vi "Calculate Source Voltage Array.vi"(8 "error in":errorcluster, 11 "measurement configuration":T1={"Mode of operation"=enum."Perform measurement", "DUT setup time"=1.0, "Source delay"=0.005, "Aperture time"=0.005, "Nominal output voltage"=3.3, "Source pin name array"=[], "Source pin name index for efficiency"=0, "Source sense array"=[], "Source current limit array"=[], "Source maximum power array"=[], "Source start voltage array"=[], "Source stop voltage array"=[], "Source voltage sweep points"=10, "Use Source voltage array"=FALSE, "Source voltage concatenated array"=[], "Source voltage array size"=[], "Load pin name"="", "Load sense"=1009, "Load voltage limit range"=6.0, "Load sweep type"="Logarithmic", "Load start current"=0.1, "Load stop current"=24.0, "Load current sweep points/points per decade"=10, "Use Load current array"=FALSE, "Load current array"=[], "Pin Names for Scope"=[], "vertical range"=[], "vertical offset"=[], "probe attenuation"=[], "vertical coupling"=[], "channel enabled"=[], "input impedance"=[], "max input frequency"=[], "min sample rate"=[], "reference position"=[], "min record length"=[], "enforce realtime"=[], "dmm pin names"=[], "dmm function array"=[], "dmm resolution in digits array"=[], "dmm range array"=[]} {"Source sense array" items=["Local"=1008, "Remote"=1009]; "dmm resolution in digits array" items=["3 1/2"=3.5, "4 1/2"=4.5, "5 1/2"=5.5, "6 1/2"=6.5, "7 1/2"=7.5]; "input impedance" items=["1 mega ohm"=0, "50 ohms"=2]; "vertical coupling" items=["AC", "DC", "Ground"]; "Load sense" items=["Local"=1008, "Remote"=1009]}) -> (0 "error out":errorcluster, 2 "Source voltage array size":i32[](array[numeric]), 3 "Source voltage array":dbl[][](array[numeric]))   [LabVIEW 2021, in "Efficiency And Load Regulation with Pin Map.lvlib"]
uses:
  Efficiency And Load Regulation with Pin Map.lvlib
  Measurement Configuration.ctl
  <instrlib>/niScope/Controls/niScope vertical coupling.ctl
  <instrlib>/niDMM/nidmm.llb/niDMM Function.ctl
  <instrlib>/niDMM/nidmm.llb/niDMM Resolution in Digits.ctl
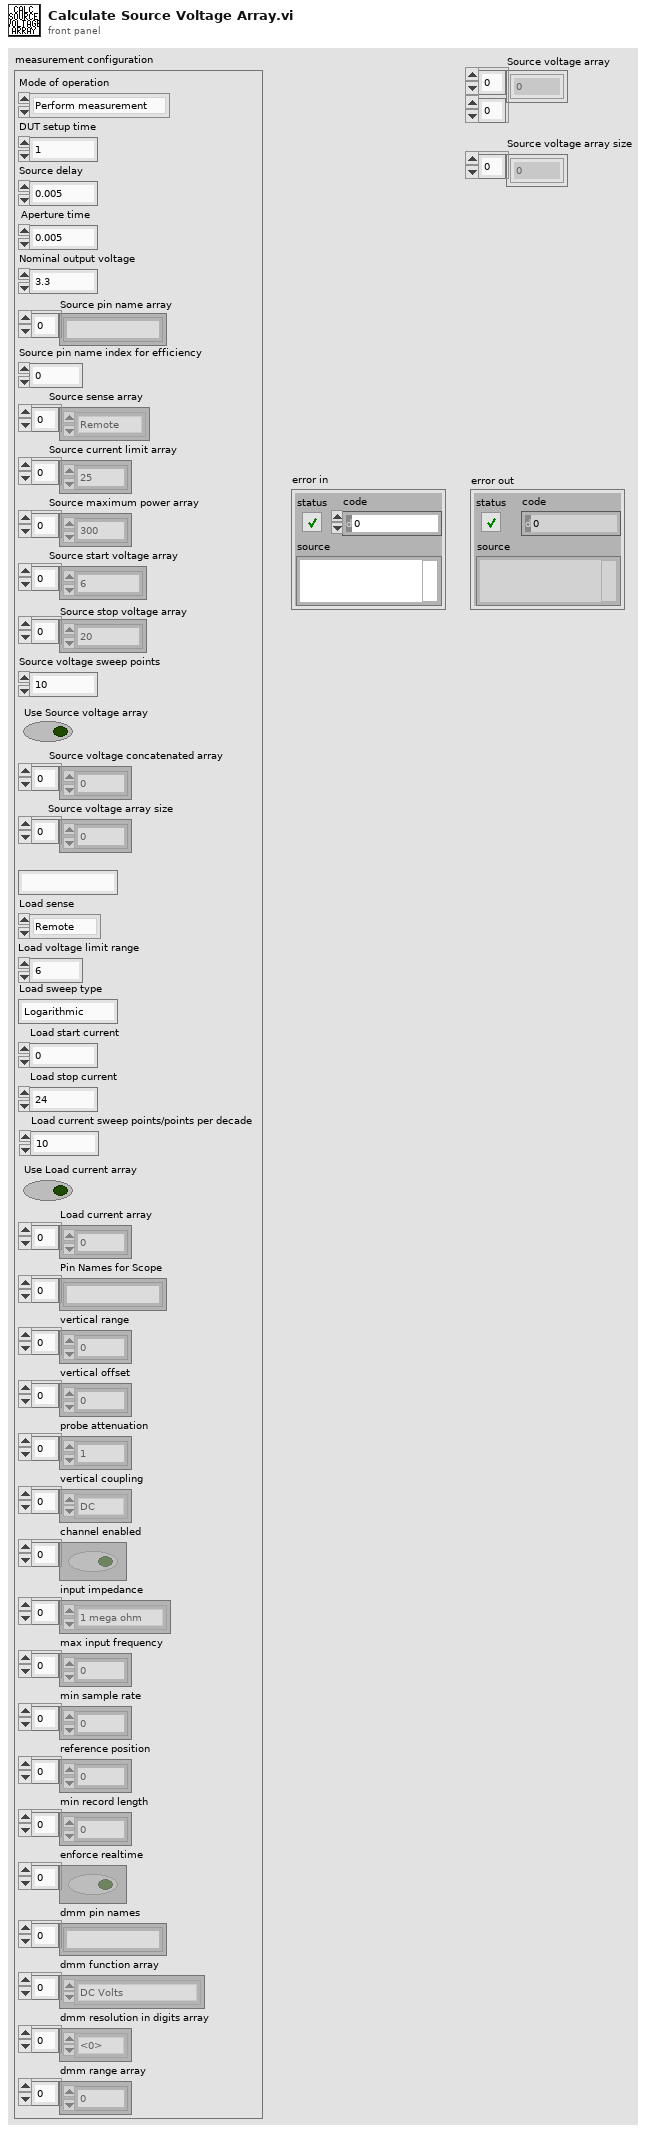
[diagram p1: front panel]
types:
  T1 = typedef "Efficiency And Load Regulation with Pin Map.lvlib/Measurement Configuration.ctl" = cluster{"Mode of operation":enum32{"Power on the DUT", "Perform measurement", "Power off the DUT"}, "DUT setup time":dbl, "Source delay":dbl, "Aperture time":dbl, "Nominal output voltage":dbl, "Source pin name array":string[], "Source pin name index for efficiency":i32, "Source sense array":i32[], "Source current limit array":dbl[], "Source maximum power array":dbl[], "Source start voltage array":dbl[], "Source stop voltage array":dbl[], "Source voltage sweep points":i32, "Use Source voltage array":bool, "Source voltage concatenated array":dbl[], "Source voltage array size":i32[], "Load pin name":string, "Load sense":i32, "Load voltage limit range":dbl, "Load sweep type":string, "Load start current":dbl, "Load stop current":dbl, "Load current sweep points/points per decade":i32, "Use Load current array":bool, "Load current array":dbl[], "Pin Names for Scope":string[], "vertical range":dbl[], "vertical offset":dbl[], "probe attenuation":dbl[], "vertical coupling":T2[], "channel enabled":bool[], "input impedance":u32[], "max input frequency":dbl[], "min sample rate":dbl[], "reference position":dbl[], "min record length":i32[], "enforce realtime":bool[], "dmm pin names":string[], "dmm function array":T3[], "dmm resolution in digits array":T4[], "dmm range array":dbl[]}
  T2 = typedef "niScope vertical coupling.ctl" = i32
  T3 = typedef "niDMM Function.ctl" = enum16{"DC Volts", "AC Volts", "DC Current", "AC Current", "2-wire Resistance", "4-wire Resistance", "Diode", "Frequency", "Period", "AC Volts DC Coupled", "Capacitance", "Inductance", "Temperature"}
  T4 = typedef "niDMM Resolution in Digits.ctl" = dbl
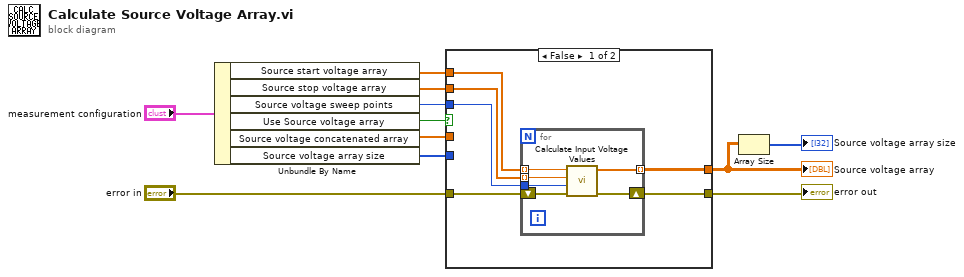
[diagram p0: block diagram]
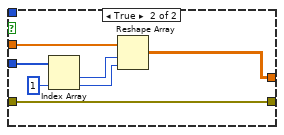
[diagram p2: hidden frame]
diagram:
  n1 = Unbundle By Name("measurement configuration") -> ("Source start voltage array"=w6:dbl[], "Source stop voltage array"=w7:dbl[], "Source voltage sweep points"=w8:i32, "Use Source voltage array"=w10:bool, "Source voltage concatenated array"=w9:dbl[], "Source voltage array size"=w1:i32[])
  n2 = case shown="False" w10 {
    tunnel: w9 -> [_ w29]
    tunnel: w8 -> [w15 _]
    tunnel: w7 -> [w16 _]
    tunnel: w6 -> [w17 _]
    tunnel: [w14 w24] -> w3
    tunnel: "error in" -> [w13 w30]
    tunnel: [w12 w30] -> w4
    tunnel: w1 -> [_ w28]
    frame False {
      n3 = for {
        tunnel: w17 -> [w23] mode=indexing
        tunnel: w16 -> [w22] mode=indexing
        tunnel: w15 -> [w21]
        tunnel: [w20] -> w14 mode=indexing
        shift-right: [w18] -> w12
        shift-left: w13 -> [w19]
        n4 = call "Calculate Input Voltage Values.vi"("error in"=w19, "Points"=w21, "Voltage stop level"=w22, "Voltage start level"=w23) -> ("error out"=w18:errorcluster, "Voltage values"=w20:dbl[])  [unwired: 6 in]
      }
    }
    frame True {
      n5 = Index Array(array=w28, index #2=1 ("index")) -> (element #1=w26:i32, element #2=w25:i32)  [unwired: 1 in]
      n6 = Reshape Array(w29, w26, w25) -> (w24:dbl[][])
    }
  }
  "error out" <- w4
  "Source voltage array" <- w3
  n7 = Array Size(array=w3) -> (size(s)=→"Source voltage array size":i32[])
